vi "Import Configuration File.vi"(8 "error in":errorcluster, 9 "include direction section?":bool, 10 "parameters configuration file path":path caption="path to parameters xml", 11 "custom device":T1 format="%.0x") -> (0 "error out":errorcluster, 3 "custom device out":T1 format="%.0x")   [LabVIEW 2020, in "AIM MIL-STD-1553 Scripting.lvlib"]
doc: "For the specified <b>custom device</b>, imports the Parameters Configuration File located at the input <b>parameters configuration file path</b>."
uses:
  AIM MIL-STD-1553 Scripting.lvlib
  <vilib>/NI VeriStand/Custom Device API/Custom Device Item Ref.ctl
  Import/MIL-STD 1553 Import.lvlib
  <vilib>/NI VeriStand/Custom Device API/Custom Device API.lvlib
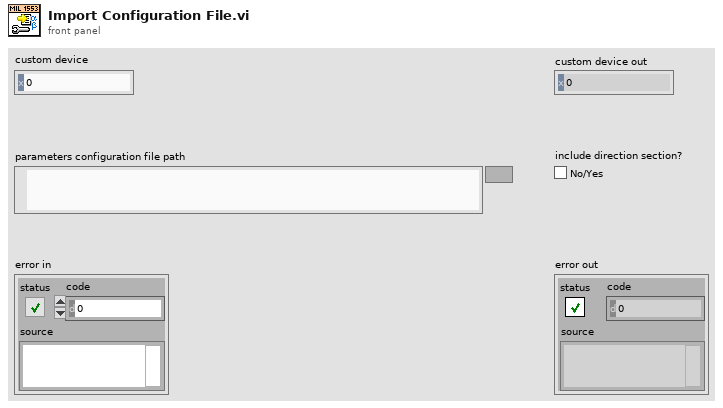
[diagram p1: front panel]
types:
  T1 = typedef "Custom Device API.lvlib/Custom Device Item Ref.ctl" = u64
  T2 = typedef "BIU Configuration.ctl" = cluster{"HW channel":u16, "terminal addresses":T3[], "terminal names":string[], "major frames":T4[], "minor frames":T5[], "acyclic frames":T6[], "messages":T7[], "minor frame period (us)":i32, "starting buffer index":u16}
  T3 = typedef "Address.ctl" = u16
  T4 = typedef "Major Frame Definition.ctl" = cluster{"name":string, "minor frames":string[]}
  T5 = typedef "Minor Frame Definition.ctl" = cluster{"name":string, "messages":string[]}
  T6 = typedef "Acyclic Frame Definition.ctl" = cluster{"name":string, "messages":string[]}
  T7 = typedef "Message Definition.ctl" = cluster{"name":string, "message type":T8, "endpoint Tx":T9, "endpoint Rx":T9, "create timestamp channel":bool, "mode code":u16, "number of words":u16, "parameters":cluster{"name":string, "default value":dbl, "unit":string, "parameter definition":T10}[]}
  T8 = typedef "Message Type.ctl" = string
  T9 = typedef "Terminal Endpoint.ctl" = cluster{"terminal address":T3, "subaddress":T3}
  T10 = typedef "Parameter Definition.ctl" = cluster{"start index":i32, "size (bits)":i32, "encoding":enum16{"BNR", "BCD", "Discrete"}, "signed":bool, "multiplier":dbl, "offset":dbl}
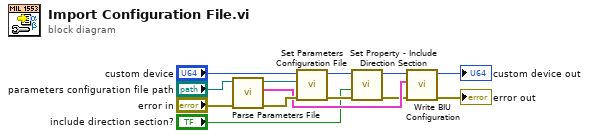
[diagram p0: block diagram]
diagram:
  n1 = call "Parse Parameters File.vi"("error in"="error in", "path to XML document"="parameters configuration file path") -> ("error out"=w12:errorcluster, "biu configuration"=w6:T2, "path to XML document out"=w13:path)  [unwired: 7 in]
  n2 = call "Set Parameters Configuration File.vi"("error in"=w12, "parameters configuration file path"=w13, "custom device"="custom device") -> ("error out"=w3:errorcluster, "custom device out"=w5:T1)  [unwired: 7 in]
  n3 = call "Set Property - Include Direction Section.vi"("error in"=w3, "include direction section"="include direction section?", "custom device"=w5) -> ("error out"=w2:errorcluster, "custom device out"=w4:T1)  [unwired: 7 in]
  n4 = call "Write BIU Configuration.vi"("error in"=w2, "biu configuration"=w6, "custom device"=w4) -> ("error out"=→"error out":errorcluster, "custom device out"=→"custom device out":T1)  [unwired: 7 in]
